vi "DependencyChecker_Example1.vi"() -> ()   [LabVIEW 2020]
uses:
  <resource>/Framework/Providers/Open_GDS/DependencyViewer/DependencyChecker/LibraryDependentInfo.vi
  <vilib>/Utility/lvfile.llb/FT_FileTypes.ctl
  <resource>/Framework/Providers/Open_GDS/DependencyViewer/DependencyChecker/FilterOptions.ctl
  <resource>/Framework/Providers/Open_GDS/DependencyViewer/DependencyChecker/DependencyChecker.lvlib
  <resource>/Framework/Providers/Open_GDS/DependencyViewer/VISJS-Viewer/VISJS Viewer.lvlib
  <vilib>/Utility/lvfile.llb/NI_FileType.lvlib
panel:
  in  "Some Filtering Options":T1(ring)=enum."Only Classes"
  out "LibraryDependencies":map{path, T2}(c390)
  in  "File Path":path=path "vi.lib/AppBuilder"
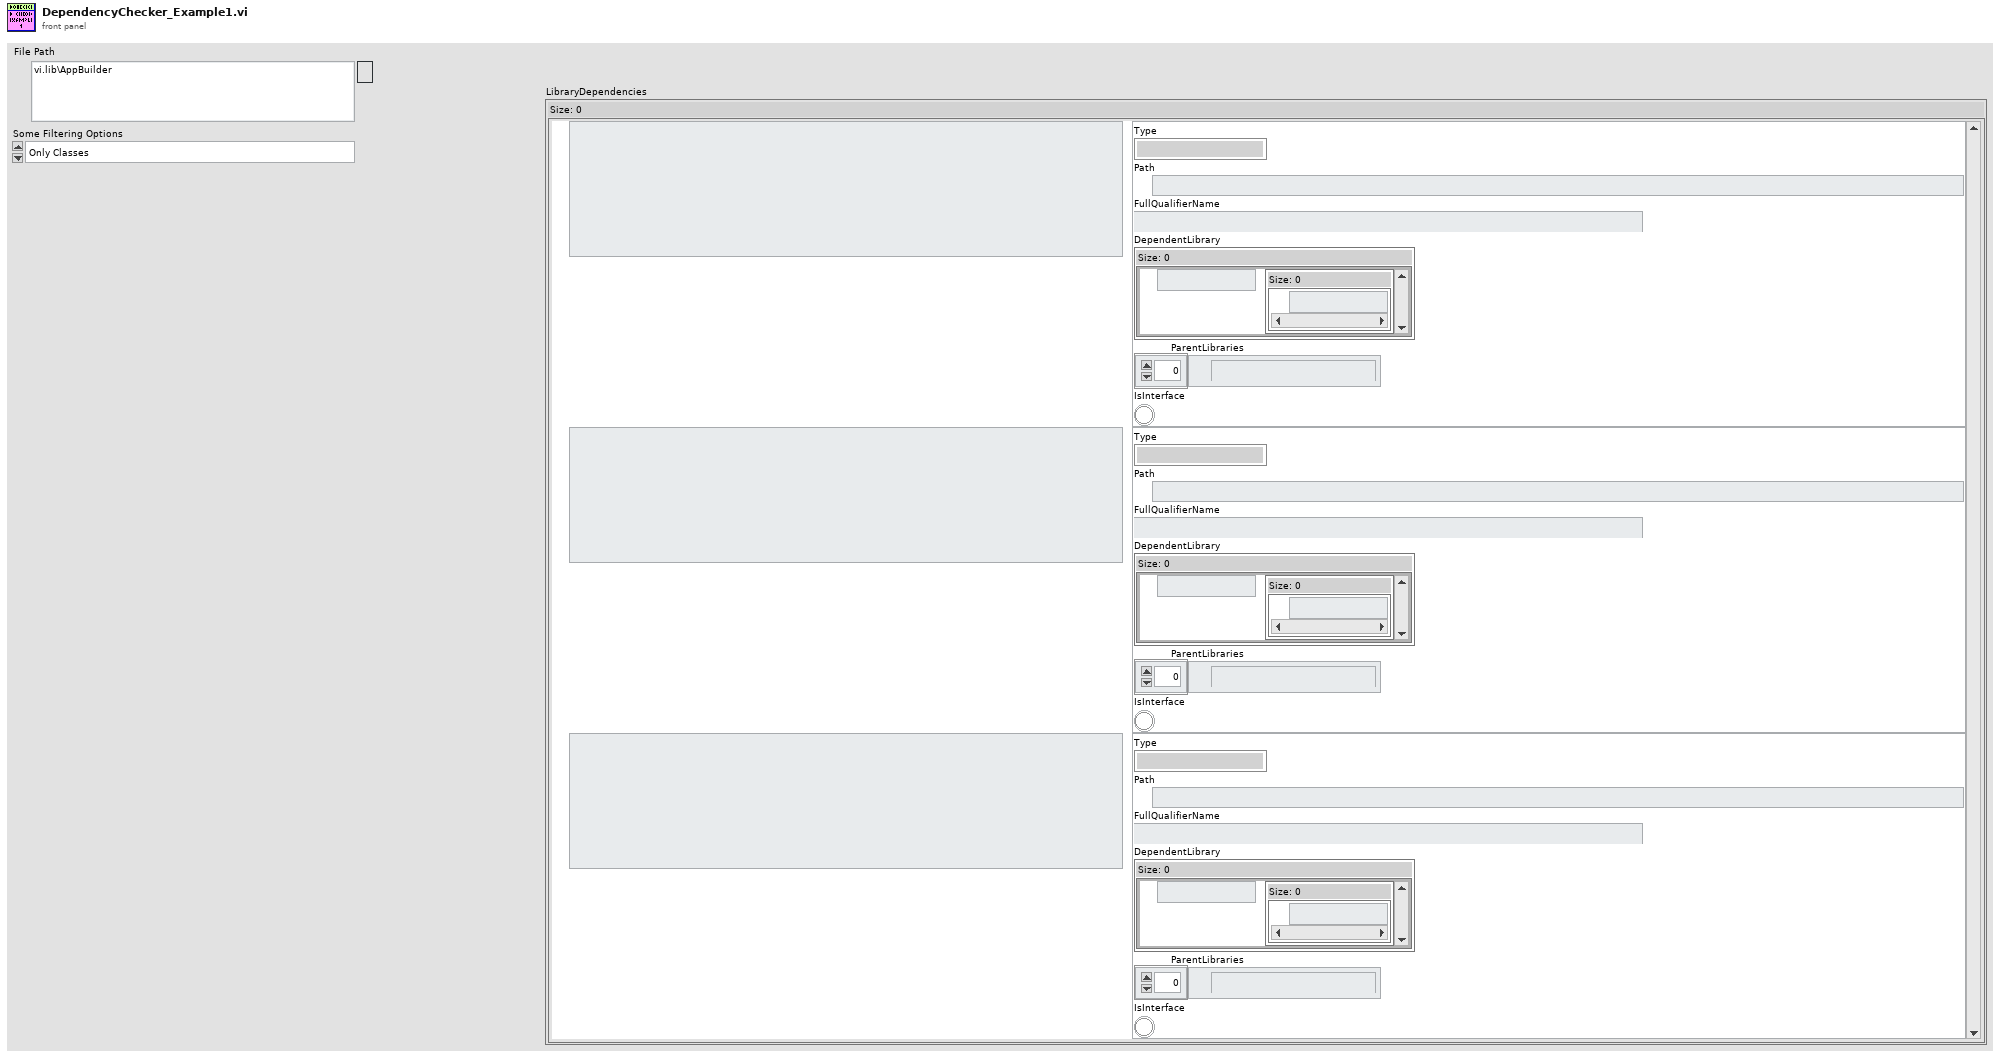
[diagram p1: front panel]
types:
  T1 = enum16{"All Classes and Libraries", "Libraries and Classes not belonging to any library", "Only Classes", "Only Libraries", "Only Libraries (no sub libraries)", "Only Items with Circular Dependencies", "Only Classes with Circular Dependencies", "Only Libraries with Circular Dependencies"}
  T2 = typedef "DependencyChecker.lvlib/LibraryDependentInfo.vi" = cluster{"Type":T3, "Path":path, "FullQualifierName":string, "DependentLibrary":map{path, set{path}}, "ParentLibraries":path[], "IsInterface":bool}
  T3 = typedef "NI_FileType.lvlib/FT_FileTypes.ctl" = enum32{"Invalid file/path", "Unknown type", "Instrument", "Control", "Polymorphic VI", "Project", "Library", "LVClass", "XControl", "XNode", "CIN", "Run-time menu", "Palette menu", "LLB", "Shortcut", "Directory", "Class Private Data Control", "Statechart", "MathScript .m file", "Ladder Diagram", "LVLibp"}
  T4 = typedef "DependencyChecker.lvlib/FilterOptions.ctl" = cluster{"Ignore user.lib":bool, "Ignore vi.lib":bool, "Ignore instr.lib":bool, "FolderToIgnore":path[], "Ignore libraries":bool, "Ignore lvcasses":bool, "Ignore xnodes":bool, "Ignore xcontrols":bool, "Ignore Channel Classes":bool}
  T5 = typedef "DependencyChecker.lvlib/FileDependencyType.ctl" = cluster{"Path":path, "FileType":T3, "FullQualifierName":string, "OwnerPath":path, "Dependencies":path[], "ParentLibraries":path[], "IsInterface":bool}
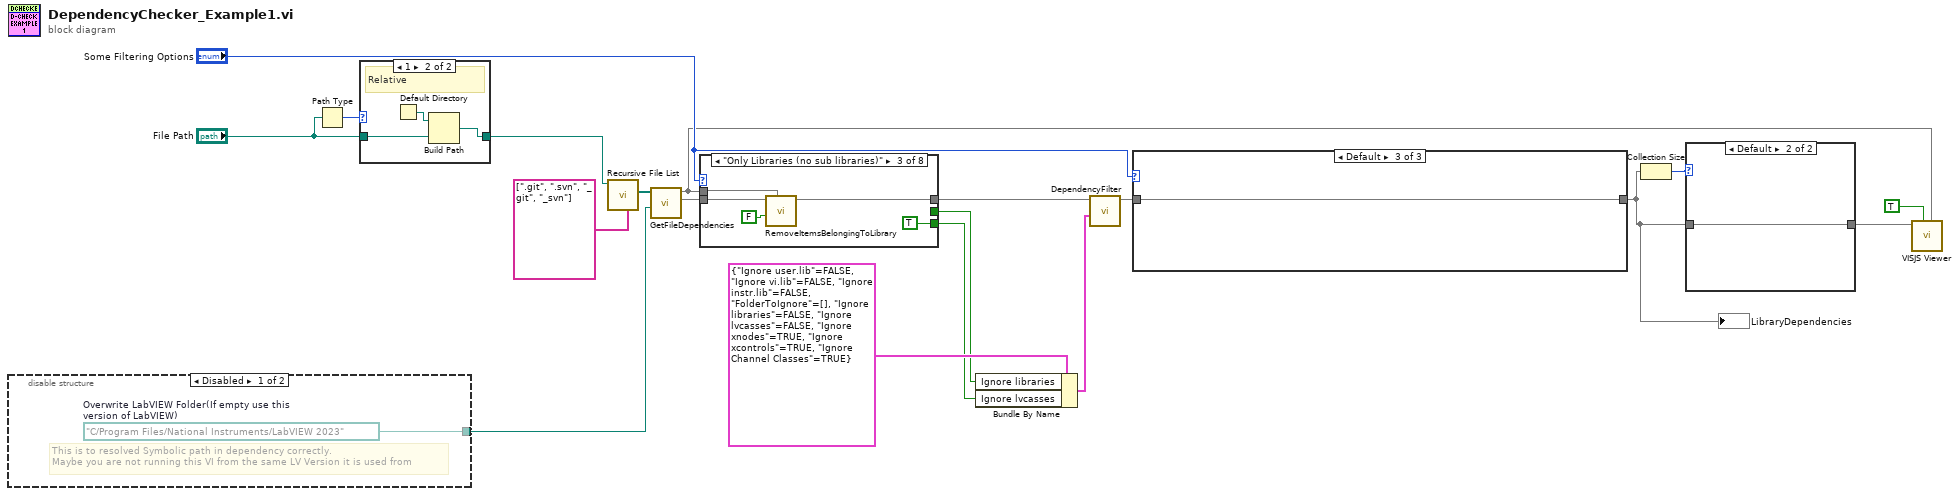
[diagram p0: block diagram]
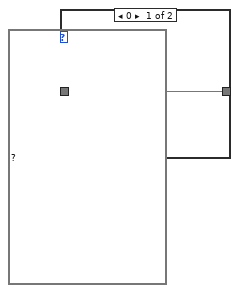
[diagram p2: hidden frame]
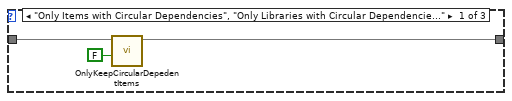
[diagram p3: hidden frame]
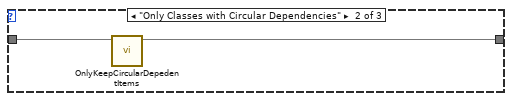
[diagram p4: hidden frame]
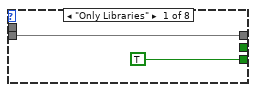
[diagram p6: hidden frame]
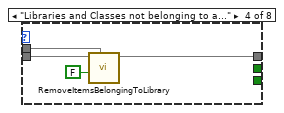
[diagram p8: hidden frame]
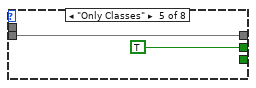
[diagram p9: hidden frame]
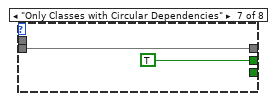
[diagram p11: hidden frame]
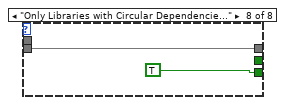
[diagram p12: hidden frame]
diagram:
  n1 = disable-structure shown="Disabled" {
    disable-tunnel: [w20 _] -> w16
    frame Disabled {
      w20 = path "C:/Program Files/National Instruments/LabVIEW 2023"  # Overwrite LabVIEW Folder(If empty use this version of LabVIEW)
      # "This is to resolved Symbolic path in dependency correctly.\nMaybe you are not running this VI from the same LV Version it is used from"
    }
    frame Enabled {
    }
  }
  n2 = Path Type(1:"File Path") -> (0:w9:i16)
  n3 = case shown="1" w9 {
    tunnel: "File Path" -> [w21 w23]
    tunnel: [w21 w22] -> w7
    frame 0, Default {
      # "Absolute Path"
    }
    frame 1 {
      # "Relative"
      n4 = Default Directory() -> (w24:path)
      n5 = Build Path(base path=w24, name or relative path=w23) -> (appended path=w22:path)
    }
  }
  n6 = call <vilib>:"Recursive File List.vi"("Folders to Exclude"=string[] [".git", ".svn", "_git", "_svn"], "Folder Path"=w7) -> ("All Files in Dir"=w19:path[])  [unwired: 5 in, 4 out]
  n7 = call <resource>:"GetFileDependencies.vi"("Overwrite LabVIEW Folder(If empty use this version of LabVIEW)"=w16, "All Files in Dir"=w19) -> ("LibraryDependency"=w15:map{path, T2}, "FileDependency out"=w1:map{path, T5})  [unwired: 8 in]
  n8 = case shown="\"Only Libraries (no sub libraries)\"" "Some Filtering Options" {
    tunnel: [w26 w27 w30 w34 w38 w39 w40 w42] -> w14
    tunnel: w15 -> [w26 w27 w32 w36 w38 w39 w40 w42]
    tunnel: [_ _ _ _ TRUE _ TRUE _] -> w11
    tunnel: [TRUE _ TRUE _ _ _ _ TRUE] -> w10
    tunnel: w1 -> [_ _ w28 w33 _ _ _ _]
    frame "Only Libraries" {
    }
    frame "All Classes and Libraries" {
    }
    frame "Only Libraries (no sub libraries)" {
      n9 = call <resource>:"RemoveItemsBelongingToLibrary.vi"("FileDependency In"=w28, "EvenSubLibraries"=FALSE, "LibraryDependency In"=w32) -> ("LibraryDependency Out"=w30:map{path, T2})  [unwired: 8 in]
    }
    frame "Libraries and Classes not belonging to any library" {
      n10 = call <resource>:"RemoveItemsBelongingToLibrary.vi"("FileDependency In"=w33, "EvenSubLibraries"=FALSE, "LibraryDependency In"=w36) -> ("LibraryDependency Out"=w34:map{path, T2})  [unwired: 8 in]
    }
    frame "Only Classes" {
    }
    frame "Only Items with Circular Dependencies" {
    }
    frame "Only Classes with Circular Dependencies" {
    }
    frame "Only Libraries with Circular Dependencies" {
    }
  }
  n11 = Bundle By Name(cluster=T4 {"Ignore user.lib"=FALSE, "Ignore vi.lib"=FALSE, "Ignore instr.lib"=FALSE, "FolderToIgnore"=[], "Ignore libraries"=FALSE, "Ignore lvcasses"=FALSE, "Ignore xnodes"=TRUE, "Ignore xcontrols"=TRUE, "Ignore Channel Classes"=TRUE} ("FilterOptions"), "Ignore libraries"=w11, "Ignore lvcasses"=w10) -> (w13:T4)
  n12 = call <resource>:"DependencyFilter.vi"("FilterOptions"=w13, "LibraryDependency In"=w14) -> ("Filtered LibraryDependency Out"=w6:map{path, T2})  [unwired: 9 in]
  n13 = case shown="Default" "Some Filtering Options" {
    tunnel: [w45 w47 w49] -> w2
    tunnel: w6 -> [w46 w48 w49]
    frame "Only Items with Circular Dependencies", "Only Libraries with Circular Dependencies" {
      n14 = call <resource>:"OnlyKeepCircularDepedentItems.vi"("IgnoreLibrariesInCircularDependencies(True)"=FALSE, "LibraryDependency In"=w46) -> ("LibraryDependency Out"=w45:map{path, T2})  [unwired: 9 in]
    }
    frame "Only Classes with Circular Dependencies" {
      n15 = call <resource>:"OnlyKeepCircularDepedentItems.vi"("LibraryDependency In"=w48) -> ("LibraryDependency Out"=w47:map{path, T2})  [unwired: 10 in]
    }
    frame Default {
    }
  }
  "LibraryDependencies" <- w2
  n16 = Collection Size(1:w2) -> (0:w4:i32)
  n17 = case shown="Default" w4 {
    tunnel: [map{path, T2} {} ("map") w51] -> w3
    tunnel: w2 -> [_ w51]
    frame 0 {
    }
    frame Default {
    }
  }
  n18 = call <resource>:"VISJS Viewer.vi"("FileDependency In"=w1, "OpenWebBrowser(False)"=TRUE, "LibraryDependency"=w3) -> ()  [unwired: 7 in, 2 out]
